vi "Play Path.vi"(4 "Align for Path":bool, 5 "Right Setpoint (Turning)":dbl, 6 "Synchronication":enum16{"Start", "Wait"}(ring), 7 "Description":string, 8 "Command Info In":T1, 9 "Reverse (T) / Normal (F)":bool, 10 "Path Reversed":bool, 11 "Path":path) -> (0 "Command Info Out":T1)   [LabVIEW 2018]
doc: "This VI notifies the subsystem to the new setpoint."
uses:
  <vilib>/Rock Robotics/WPI/Framework/Command Status Info.ctl
  <vilib>/Rock Robotics/WPI/Framework/Completion Status.ctl
  <vilib>/Rock Robotics/WPI/Framework/Completion Notifier.ctl
  Support Code/Availible Command systems for auto.ctl
  Implementation/Drive Operations.ctl
  Implementation/Drive Setpoints.ctl
  Support Code/Path Data.ctl
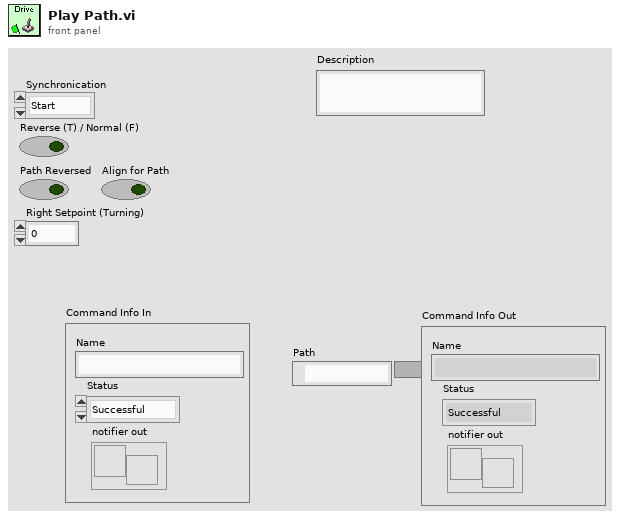
[diagram p1: front panel]
types:
  T1 = typedef "Command Status Info.ctl" = cluster{"Name":string, "Status":T2, "notifier out":T3}
  T2 = typedef "Completion Status.ctl" = enum16{"Successful", "Aborted", "Incomplete"}
  T3 = typedef "Completion Notifier.ctl" = refnum<notifier>
  T4 = typedef "Availible Command systems for auto.ctl" = u16
  T5 = cluster{"V":dbl[], "Theta":dbl[], "Commands":cluster{"Time into Path":dbl, "System":T4, "Item Selected?":bool, "System Selection":T4}[], "Sample Period":dbl}
  T6 = typedef "Drive Operations.ctl" = enum16{"Reserve", "Read Current", "Immediate", "J-Turn", "Play Back From Log", "Auto-Align"}
  T7 = typedef "Drive Setpoints.ctl" = cluster{"Operation":T6, "Left Setpoint (Power)":dbl, "Right Setpoint (Turning)":dbl, "Reverse (T) / Normal (F)":bool, "Power Scaling (1=Normal) ":dbl, "Path Data":T8, "Path":path, "Angle boi":dbl, "Path Reversed":bool, "Align for Path":bool, "80A(T)/45(F)":bool, "Auto Path Data":cluster{"V":dbl[], "Theta":dbl[], "Commands":cluster{"Time into Path":dbl, "System":T4, "Item Selected?":bool, "System Selection":T4}[], "Sample Period":dbl}}
  T8 = typedef "Path Data.ctl" = cluster{"Maneuver":enum16{"MAX 90", "MAX 180", "Turn to Home", "Turn to Rocket", "Auto-Align", "Turn to ..."}, "Rotation Direction":enum16{"N/A", "Right", "Left"}}[]
  T9 = cluster{"Segment Name":string, "Type":enum16{"Accel Straight", "Const Straight", "Blend", "Circle"}, "Traj Pos Points":cluster{"x":dbl, "y":dbl, "th":dbl}[], "Traj Vel Points":cluster{"V":dbl, "th":dbl}[], "Accel Index":i32, "Decel Index":i32}[]
  T10 = cluster{"Time into Path":dbl, "System":T4, "Item Selected?":bool, "System Selection":T4}[]
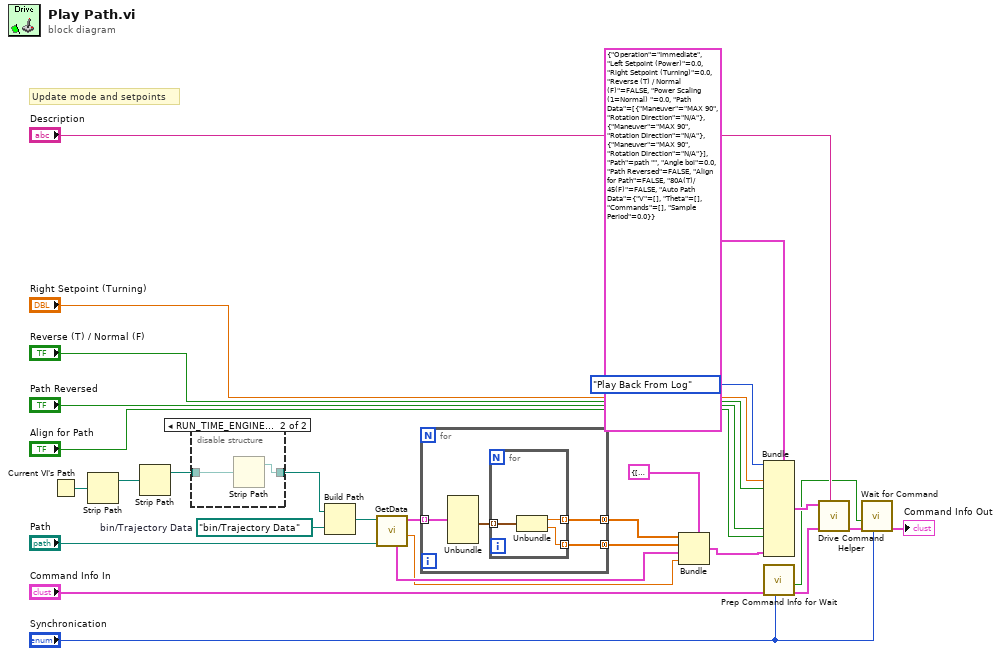
[diagram p0: block diagram]
diagram:
  w10 = path "bin/Trajectory Data"  # bin/Trajectory Data
  # "Update mode and setpoints"
  n1 = Current VI's Path() -> (path=w12:path)
  n2 = Strip Path(path=w12) -> (stripped path=w11:path)  [unwired: 1 out]
  n3 = Strip Path(path=w11) -> (stripped path=w8:path)  [unwired: 1 out]
  n4 = disable-structure shown="RUN_TIME_ENGINE==True, Default" {
    disable-tunnel: [w29 w30] -> w9
    disable-tunnel: w8 -> [w29 w31]
    frame condition #0 (active) {
    }
    frame condition #1 {
      n5 = Strip Path(path=w31) -> (stripped path=w30:path)  [unwired: 1 out]
    }
  }
  n6 = Build Path(base path=w9, name or relative path=w10) -> (appended path=w13:path)
  n7 = call "GetData.vi"("File"="Path", "file (use dialog)"=w13) -> ("Sample Period (s)"=w2:dbl, "Trajectory Data"=w14:T9, "Commands"=w4:T10)  [unwired: 2 in, 5 out]
  n8 = for {
    tunnel: [w35] -> w7 mode=concatenating
    tunnel: [w34] -> w6 mode=concatenating
    tunnel: w14 -> [w32] mode=indexing
    n9 = Unbundle(w32) -> ("Traj Vel Points"=w33:cluster{"V":dbl, "th":dbl}[])  [unwired: 5 out]
    n10 = for {
      tunnel: w33 -> [w36] mode=indexing
      tunnel: [w38] -> w35 mode=indexing
      tunnel: [w37] -> w34 mode=indexing
      n11 = Unbundle(w36) -> ("V"=w38:dbl, "th"=w37:dbl)
    }
  }
  n12 = Bundle(cluster=T5 {"V"=[], "Theta"=[], "Commands"=[], "Sample Period"=0.0} ("Auto Path Data"), "V"=w7, "Theta"=w6, "Commands"=w4, "Sample Period"=w2) -> (w1:T5)
  n13 = Bundle(cluster=T7 {"Operation"=enum."Immediate", "Left Setpoint (Power)"=0.0, "Right Setpoint (Turning)"=0.0, "Reverse (T) / Normal (F)"=FALSE, "Power Scaling (1=Normal) "=0.0, "Path Data"=[{"Maneuver"=enum."MAX 90", "Rotation Direction"=enum."N/A"}, {"Maneuver"=enum."MAX 90", "Rotation Direction"=enum."N/A"}, {"Maneuver"=enum."MAX 90", "Rotation Direction"=enum."N/A"}], "Path"=path "", "Angle boi"=0.0, "Path Reversed"=FALSE, "Align for Path"=FALSE, "80A(T)/45(F)"=FALSE, "Auto Path Data"={"V"=[], "Theta"=[], "Commands"=[], "Sample Period"=0.0}} ("SubSystem Data"), "Operation"=Drive_Operations."Play Back From Log", "Right Setpoint (Turning)"="Right Setpoint (Turning)", "Reverse (T) / Normal (F)"="Reverse (T) / Normal (F)", "Path Reversed"="Path Reversed", "Align for Path"="Align for Path", "Auto Path Data"=w1) -> (w26:T7)  [unwired: 6 in]
  n14 = call <vilib>:"Prep Command Info for Wait.vi"("Synchronication"="Synchronication", "Command Info"="Command Info In") -> ("Command Info"=w24:T1, "Allocated"=w20:bool)  [unwired: 8 in]
  n15 = call "Drive Command Helper.vi"("Description"="Description", "Command Info In"=w24, "SubSystem Data"=w26) -> ("Command Info Out"=w23:T1)  [unwired: 6 in, 2 out]
  n16 = call <vilib>:"Wait for Command.vi"("Synchronication"="Synchronication", "Command Info in"=w23, "Allocated"=w20) -> ("Command Info out"=→"Command Info Out":T1)  [unwired: 8 in]
